vi "ISEG_HVChannel.update services and attribute data.vi"(0 "i ref in":refnum<vi>, 1 "direction":T3=enum."update actual value", 2 "service":T2, 3 "ms timeout (10000)":i32=10000, 4 "value":string, 5 "error in (no error)":errorcluster, 7 "quality":T1=enum."on") -> (14 "i ref out":refnum<vi>, 17 "timed out":bool, 19 "error out":errorcluster)   [LabVIEW 2014, in "ISEG_HVChannel.lvlib"]
doc: "Updates the DIM service of the attribute \"on\" and \"ramp rate\" and updates the data of the attribute."
uses:
  ISEG_HVChannel.lvlib
  CSCore/CSApplicationBaseClasses/PSChannelBase/PSChannelBase.directionType.ctl
  CSCore/CSApplicationBaseClasses/PSChannelBase/PSChannelBase.serviceType.ctl
  CSlibraries/UtilityLib/UtilityLib.valueStatus.ctl
  CSCore/CSApplicationBaseClasses/PSChannelBase/PSChannelBase.lvlib
  CSCore/CSSystem/CoreLib/CoreLib.lvlib
  CSlibraries-extern/DimLVEvent/LVDimInterface/LVDimInterface.lvlib
  CSlibraries/UtilityLib/UtilityLib.lvlib
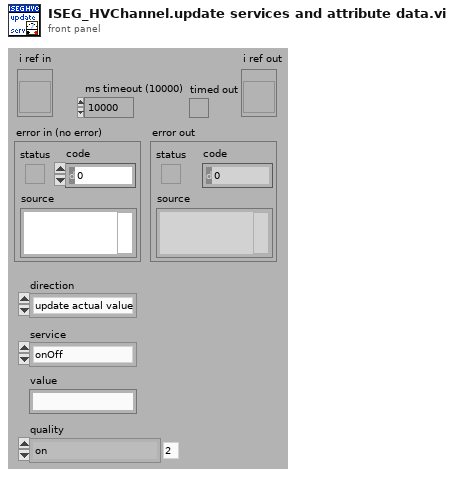
[diagram p1: front panel]
types:
  T1 = typedef "UtilityLib.lvlib/UtilityLib.valueStatus.ctl" = enum16{"no info available", "stand by/off", "on", "warning", "alarm/malfunction", "not implemented", "user action required", "important information", "system default", "control default", "indicator default", "button default"}
  T2 = typedef "PSChannelBase.lvlib/PSChannelBase.serviceType.ctl" = enum16{"onOff", "voltage", "current", "tripCurrent", "rampUpSpeed", "rampDownSpeed", "status"}
  T3 = typedef "PSChannelBase.lvlib/PSChannelBase.directionType.ctl" = enum16{"unknown", "update actual value", "update nominal value", "update both"}
  T4 = typedef "PSChannelBase.lvlib/PSChannelBase.i attribute.ctl" = cluster{"defaultChannelIndex":i32, "nofChannels":i32, "defaultChannelIndexID":i32, "nofChannelsID":i32, "actValues":T5, "nomValues":T5, "logicalName":string[], "physicalName":string[], "logicalNameID":i32, "physicalNameID":i32}
  T5 = typedef "PSChannelBase.lvlib/PSChannelBase.parameters.ctl" = cluster{"onOff":bool[], "voltage":dbl[], "current":dbl[], "tripCurrent":dbl[], "rampUpSpeed":dbl[], "rampDownSpeed":dbl[], "status":i32[], "serviceIDs":cluster{"onOfflID":i32, "voltageID":i32, "currentID":i32, "tripCurrentID":i32, "rampUpSpeedID":i32, "rampDownSpeedID":i32, "statusID":i32}}
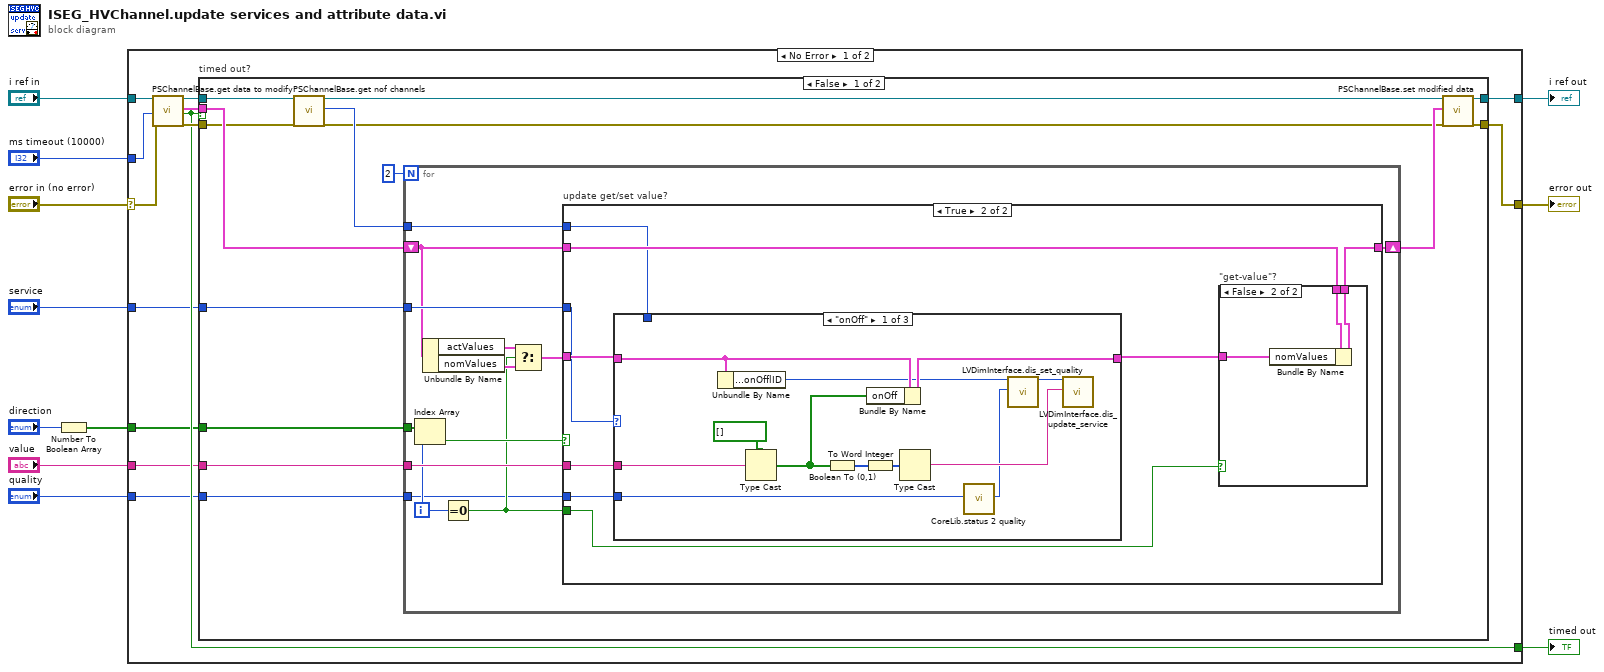
[diagram p0: block diagram]
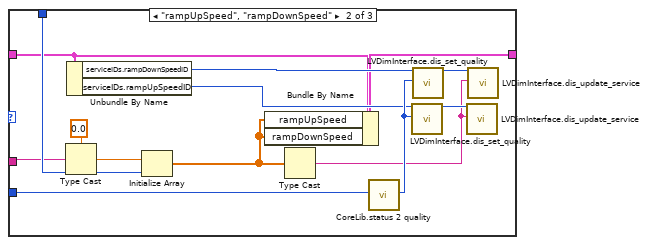
[diagram p3: hidden frame]
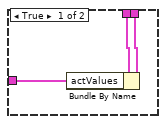
[diagram p5: hidden frame]
diagram:
  n1 = Number To Boolean Array(number="direction") -> (Boolean array=w4:bool[])
  n2 = case shown="No Error" "error in (no error)" {
    selector: "error in (no error)" -> [w22 w98]
    tunnel: [w18 w98] -> w10
    tunnel: "i ref in" -> [w24 w97]
    tunnel: [w20 w97] -> w8
    tunnel: "ms timeout (10000)" -> [w23 _]
    tunnel: [w17 _] -> w6
    tunnel: w4 -> [w15 _]
    tunnel: "service" -> [w14 _]
    tunnel: "value" -> [w13 _]
    tunnel: "quality" -> [w12 _]
    frame No Error {
      n3 = call "PSChannelBase.get data to modify.vi"("i ref in"=w24, "ms timeout (10000)"=w23, "error in (no error)"=w22) -> ("i ref out"=w21:refnum<vi>, "i attribute"=w16:T4, "timed out"=w17:bool, "error out"=w19:errorcluster)  [unwired: 13 in]
      n4 = case "timed out?" shown="False" w17 {
        tunnel: w21 -> [w29 w96]
        tunnel: [w38 w96] -> w20
        tunnel: w19 -> [w26 w95]
        tunnel: [w37 w95] -> w18
        tunnel: w16 -> [w31 _]
        tunnel: w15 -> [w36 _]
        tunnel: w14 -> [w35 _]
        tunnel: w13 -> [w34 _]
        tunnel: w12 -> [w32 _]
        frame False {
          n5 = call "PSChannelBase.get nof channels.vi"("i ref in"=w29, "error in (no error)"=w26) -> ("i ref out"=w27:refnum<vi>, "NofChannels"=w28:i32, "error out"=w25:errorcluster)  [unwired: 15 in]
          n6 = for {
            N: 2 -> [_]
            tunnel: w36 -> [w51]
            tunnel: w35 -> [w49]
            tunnel: w34 -> [w48]
            tunnel: w32 -> [w40]
            shift-right: [w41] -> w33
            shift-left: w31 -> [w43]
            tunnel: w28 -> [w39]
            i -> [w47]
            n7 = Index Array(array=w51, index=w47) -> (element=w50:bool)
            n8 = Unbundle By Name(w43) -> ("actValues"=w46:T5, "nomValues"=w45:T5)
            n9 = Equal To 0?(x=w47) -> (x = 0?=w42:bool)
            n10 = Select(t=w46, s=w42, f=w45) -> (s? t:f=w44:T5)
            n11 = case "update get/set value?" shown="True" w50 {
              tunnel: w49 -> [_ w54]
              tunnel: w48 -> [_ w60]
              tunnel: w44 -> [_ w61]
              tunnel: w43 -> [w52 w59]
              tunnel: w42 -> [_ w57]
              tunnel: [w52 w56] -> w41
              tunnel: w40 -> [_ w55]
              tunnel: w39 -> [_ w53]
              frame False {
              }
              frame True {
                n12 = case shown="\"onOff\"" w54 {
                  tunnel: w61 -> [w73 w74 w88]
                  tunnel: w60 -> [w72 w78 _]
                  tunnel: [w71 w75 w88] -> w58
                  tunnel: w55 -> [w70 w86 _]
                  tunnel: w53 -> [_ w79 _]
                  frame "onOff" {
                    n13 = Unbundle By Name(w73) -> ("serviceIDs.onOfflID"=w66:i32)
                    n14 = Type Cast(type=bool[] [] ("Boolean array"), x=w72) -> (*(type *) &x=w62:bool[])
                    n15 = Boolean To (0,1)(Boolean=w62) -> (0, 1=w64:i16[])
                    n16 = To Word Integer(number=w64) -> (16bit integer=w63:i16[])
                    n17 = Bundle By Name(cluster=w73, "onOff"=w62) -> (w71:T5)
                    n18 = Type Cast(x=w63) -> (*(type *) &x=w68:string)  [unwired: 1 in]
                    n19 = call "CoreLib.status 2 quality.vi"("valueStatus"=w70) -> ("quality"=w67:i32)  [unwired: 18 in]
                    n20 = call "LVDimInterface.dis_set_quality.vi"("my_serviceID"=w66, "quality"=w67) -> ("my_serviceID (out)"=w65:i32)  [unwired: 16 in, 1 out]
                    n21 = call "LVDimInterface.dis_update_service.vi"("my_serviceID"=w65, "data"=w68) -> ()  [unwired: 15 in, 3 out]
                  }
                  frame "rampUpSpeed", "rampDownSpeed" {
                    n22 = Type Cast(type=0.0, x=w78) -> (*(type *) &x=w80:dbl)
                    n23 = Unbundle By Name(w74) -> ("serviceIDs.rampDownSpeedID"=w83:i32, "serviceIDs.rampUpSpeedID"=w82:i32)
                    n24 = Initialize Array(w80, w79) -> (w76:dbl[])
                    n25 = Bundle By Name(cluster=w74, "rampUpSpeed"=w76, "rampDownSpeed"=w76) -> (w75:T5)
                    n26 = Type Cast(x=w76) -> (*(type *) &x=w77:string)  [unwired: 1 in]
                    n27 = call "CoreLib.status 2 quality.vi"("valueStatus"=w86) -> ("quality"=w84:i32)  [unwired: 18 in]
                    n28 = call "LVDimInterface.dis_set_quality.vi"("my_serviceID"=w82, "quality"=w84) -> ("my_serviceID (out)"=w85:i32)  [unwired: 16 in, 1 out]
                    n29 = call "LVDimInterface.dis_set_quality.vi"("my_serviceID"=w83, "quality"=w84) -> ("my_serviceID (out)"=w87:i32)  [unwired: 16 in, 1 out]
                    n30 = call "LVDimInterface.dis_update_service.vi"("my_serviceID"=w85, "data"=w77) -> ()  [unwired: 15 in, 3 out]
                    n31 = call "LVDimInterface.dis_update_service.vi"("my_serviceID"=w87, "data"=w77) -> ()  [unwired: 15 in, 3 out]
                  }
                  frame Default {
                  }
                }
                n32 = case "\"get-value\"?" shown="False" w57 {
                  tunnel: w59 -> [w91 w94]
                  tunnel: w58 -> [w90 w93]
                  tunnel: [w89 w92] -> w56
                  frame True {
                    n33 = Bundle By Name(cluster=w91, "actValues"=w90) -> (w89:T4)
                  }
                  frame False {
                    n34 = Bundle By Name(cluster=w94, "nomValues"=w93) -> (w92:T4)
                  }
                }
              }
            }
          }
          n35 = call "PSChannelBase.set modified data.vi"("i ref in"=w27, "i attribute"=w33, "error in (no error)"=w25) -> ("i ref out"=w38:refnum<vi>, "error out"=w37:errorcluster)  [unwired: 15 in]
        }
        frame True {
        }
      }
    }
    frame Error {
    }
  }
  "error out" <- w10
  "i ref out" <- w8
  "timed out" <- w6
